vi "ts_tree_set_step_results.vi"(4 "results.data":string, 6 "results.txt":string, 8 "error in (no error)":errorcluster, 9 "ts.status":bool, 10 "ts.data":T1, 11 "Tree.in":refnum<vi>) -> (0 "error out":errorcluster, 3 "Tree.out":refnum<vi>)   [LabVIEW 2015]
doc: "sets a child test step results against the current active parent tag"
uses:
  ts-data.ctl
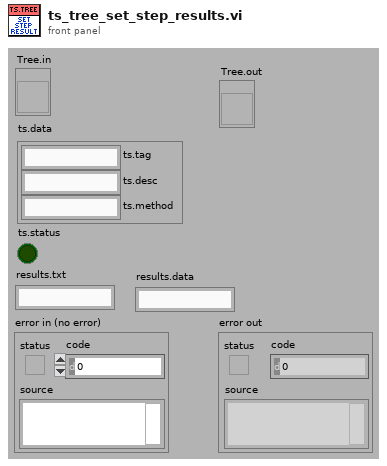
[diagram p1: front panel]
types:
  T1 = typedef "ts-data.ctl" = cluster{"ts.tag":string, "ts.desc":string, "ts.method":string}
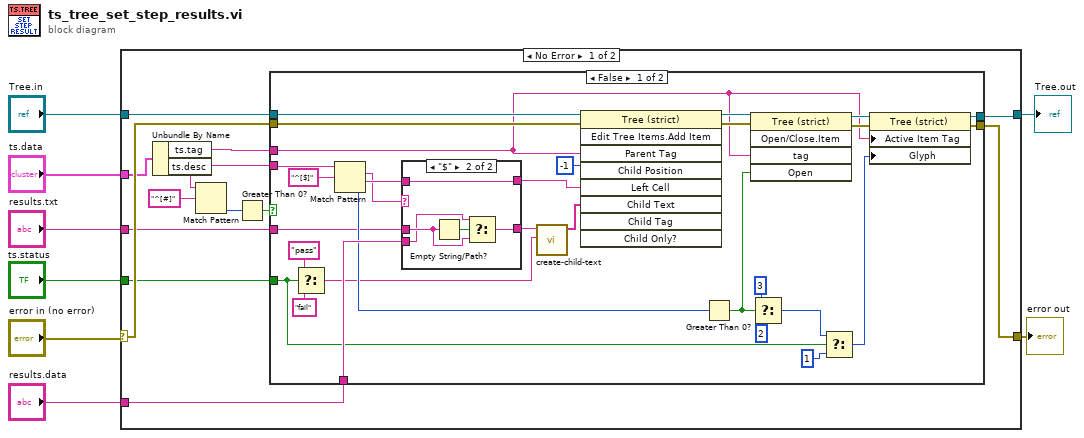
[diagram p0: block diagram]
diagram:
  n1 = case shown="No Error" "error in (no error)" {
    selector: "error in (no error)" -> [w21 w61]
    tunnel: "Tree.in" -> [w20 w62]
    tunnel: [w16 w62] -> w6
    tunnel: [w14 w61] -> w5
    tunnel: "ts.status" -> [w13 _]
    tunnel: "results.txt" -> [w19 _]
    tunnel: "ts.data" -> [w18 _]
    tunnel: "results.data" -> [w17 _]
    frame No Error {
      n2 = Unbundle By Name(w18) -> ("ts.tag"=w15:string, "ts.desc"=w9:string)
      n3 = Match Pattern(string=w9, regular expression="^[#]") -> (offset past match=w12:i32)  [unwired: 1 in, 3 out]
      n4 = Greater Than 0?(x=w12) -> (x > 0?=w10:bool)
      n5 = case shown="False" w10 {
        tunnel: w21 -> [w50 w60]
        tunnel: w20 -> [w48 w59]
        tunnel: w19 -> [w30 _]
        tunnel: w17 -> [w43 _]
        tunnel: [w41 w59] -> w16
        tunnel: w15 -> [w31 _]
        tunnel: [w40 w60] -> w14
        tunnel: w13 -> [w39 _]
        tunnel: w9 -> [w29 _]
        frame False {
          n6 = Select(t="pass", s=w39, f="fail") -> (s? t:f=w23:string)
          n7 = Match Pattern(string=w29, regular expression="^[$]") -> (match substring=w22:string, after substring=w27:string, offset past match=w36:i32)  [unwired: 1 in, 1 out]
          n8 = case shown="\"$\"" w22 {
            tunnel: w43 -> [w52 w55]
            tunnel: w30 -> [w53 w56]
            tunnel: [w53 w58] -> w28
            tunnel: w27 -> [_ w58]
            tunnel: [w52 w54] -> w25
            frame "False", Default {
            }
            frame "$" {
              n9 = Empty String/Path?(string/path=w56) -> (empty?=w57:bool)
              n10 = Select(t=w55, s=w57, f=w56) -> (s? t:f=w54:string)
            }
          }
          n11 = call "create-child-text.vi"("results.text"=w23, "results.data"=w25) -> ("Array"=w24:string[])  [unwired: 9 in]
          n12 = invoke class="Tree (strict)" method="Edit Tree Items.Add Item"(reference=w48, error in=w50, "Parent Tag"=w31, "Child Position"=-1, "Left Cell"=w28, "Child Text"=w24) -> (reference out=w47:refnum<vi>, error out=w46:errorcluster)  [unwired: 3 in, 7 out]
          n13 = Greater Than 0?(x=w36) -> (x > 0?=w26:bool)
          n14 = invoke class="Tree (strict)" method="Open/Close.Item"(reference=w47, error in=w46, "tag"=w31, "Open"=w26) -> (reference out=w42:refnum<vi>, error out=w51:errorcluster)  [unwired: 1 in, 3 out]
          n15 = Select(t=3, s=w26, f=2) -> (s? t:f=w32:i32)
          n16 = Select(t=w32, s=w39, f=1) -> (s? t:f=w37:i32)
          n17 = property class="Tree (strict)"(reference=w42, error in=w51, "Active Item Tag"=w31, "Glyph"=w37) -> (reference out=w41:refnum<vi>, error out=w40:errorcluster)
        }
        frame True {
        }
      }
    }
    frame Error {
    }
  }
  "Tree.out" <- w6
  "error out" <- w5
